vi "Query Serial Number.vi"(8 "error in":errorcluster) -> (0 "error out":errorcluster, 2 "Serial Number":string)   [LabVIEW 2009]
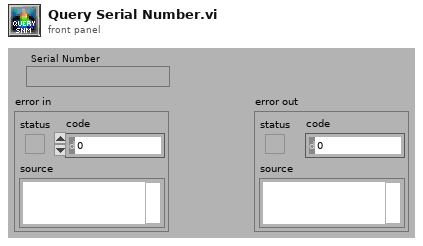
[diagram p1: front panel]
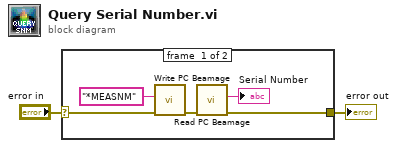
[diagram p0: block diagram]
diagram:
  n1 = case shown="No Error" "error in" {
    selector: "error in" -> [w6 w8]
    tunnel: [w3 w8] -> w1
    frame #0 {
      n2 = call "Write PC Beamage.vi"("error in"=w6, "command"="*MEASNM") -> ("error out"=w5:errorcluster)  [unwired: 9 in]
      n3 = call "Read PC Beamage.vi"("error in"=w5) -> ("error out"=w3:errorcluster, "Reply"=→"Serial Number":string)  [unwired: 9 in]
    }
    frame #1 {
    }
  }
  "error out" <- w1
